vi "Write_Wrap_Simple.vi"(4 "Value":T1) -> (1 "Var":refnum<class "Var_DBL.lvclass">)   [LabVIEW 2021, in "Var_DBL.lvclass"]
uses:
  Var_DBL.lvclass
  Type.ctl
  Var_DBL.lvclass/Var_DBL.ctl
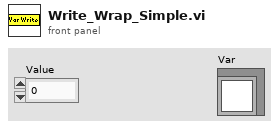
[diagram p1: front panel]
types:
  T1 = typedef "Var_DBL.lvclass/Type.ctl" = dbl
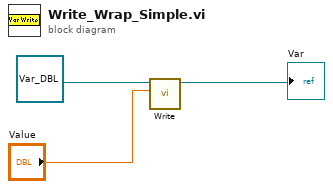
[diagram p0: block diagram]
diagram:
  n1 = call-dynamic "Write.vi"("Value"="Value", "Double Float.lvclass_340760 in"=refnum<class "Var_DBL.lvclass"> refnum ("Constants.lvlib:Numeric.lvclass")) -> ("Double Float.lvclass_340760 out"=→"Var":refnum<class "Var_DBL.lvclass">)  [unwired: 8 in, 1 out]
